vi "TraceProvisioning.vi"(8 "error in (no error)":errorcluster, 9 "addional info":string, 10 "message name":string, 11 "Qbus in":refnum<class "Qbus.lvclass">) -> (0 "error out":errorcluster, 3 "Qbus out":refnum<class "Qbus.lvclass">)   [LabVIEW 2017, in "ServerComm.lvlib"]
uses:
  <vilib>/addons/InsightCM/Devices/Shared/Common/ServerComm/ServerComm.lvlib
  <vilib>/addons/Qbus/Qbus.lvclass
  <vilib>/addons/TraceLogger/TraceLogger.lvlib
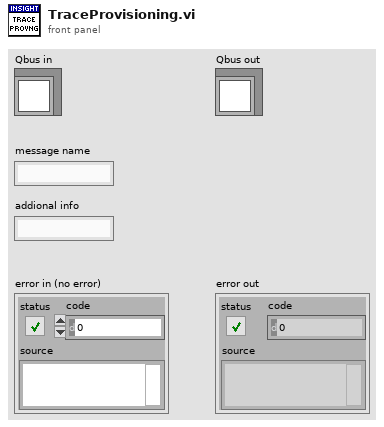
[diagram p1: front panel]
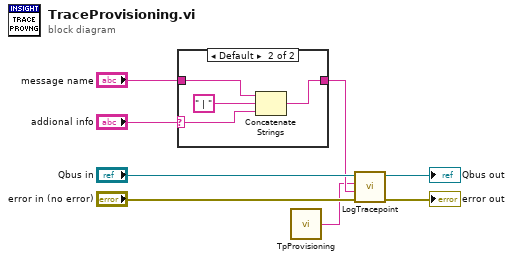
[diagram p0: block diagram]
diagram:
  n1 = case shown="Default" "addional info" {
    selector: "addional info" -> [_ w13]
    tunnel: [w9 w10] -> w4
    tunnel: "message name" -> [w9 w11]
    frame "" {
    }
    frame Default {
      n2 = Concatenate Strings(w11, " | " ("string"), w13) -> (w10:string)
    }
  }
  n3 = call <vilib>:"TpProvisioning.vi"() -> ("tracepoint name"=w1:string)  [unwired: 5 in]
  n4 = call <vilib>:"LogTracepoint.vi"("error in (no error)"="error in (no error)", "log string"=w4, "tracepoint"=w1, "qbus in"="Qbus in") -> ("error out"=→"error out":errorcluster, "qbus out"=→"Qbus out":refnum<class "Qbus.lvclass">)  [unwired: 6 in]
